vi "RT Buffered Logger.vi"(8 "error in (no error)":errorcluster, 11 "Logger Parameters":T1) -> (0 "error out":errorcluster, 3 "Logger Parameters":T1={"State"="", "Buffer size"=0, "Array Element size"=0, "Buffer Index"=0, "Data FIFO"=refnum, "is Shutdown"=FALSE, "Buffer"=[], "Log path"=path "C:/logs/AdvancedTDMS_Telemetry_Prototype.tdms", "File ref"=refnum, "Channel Names"=[]})   [LabVIEW 2019, in "Telemetry Engine.lvlib"]
uses:
  Telemetry Engine.lvlib
  Types/Logger Data.ctl
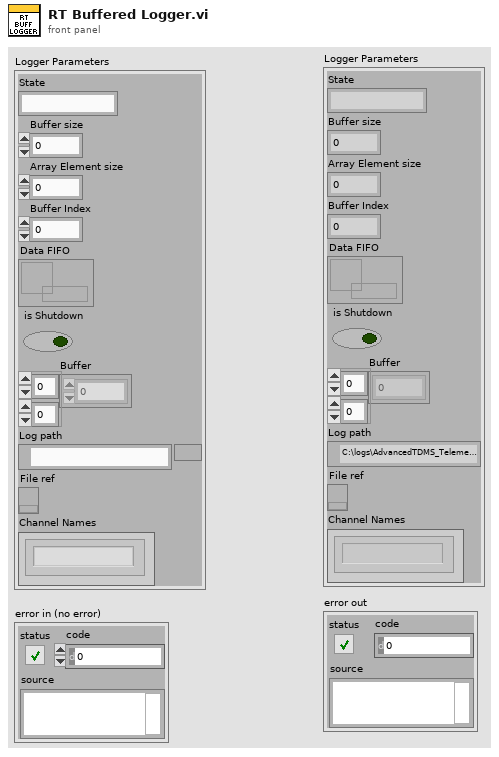
[diagram p1: front panel]
types:
  T1 = typedef "Telemetry Engine.lvlib/Logger Data.ctl" = cluster{"State":string, "Buffer size":i32, "Array Element size":i32, "Buffer Index":i32, "Data FIFO":refnum<k33>, "is Shutdown":bool, "Buffer":dbl[][], "Log path":path, "File ref":refnum<k34>, "Channel Names":string[]}
  T2 = enum16{"open", "open or create", "create or replace", "create", "open (read-only)"}
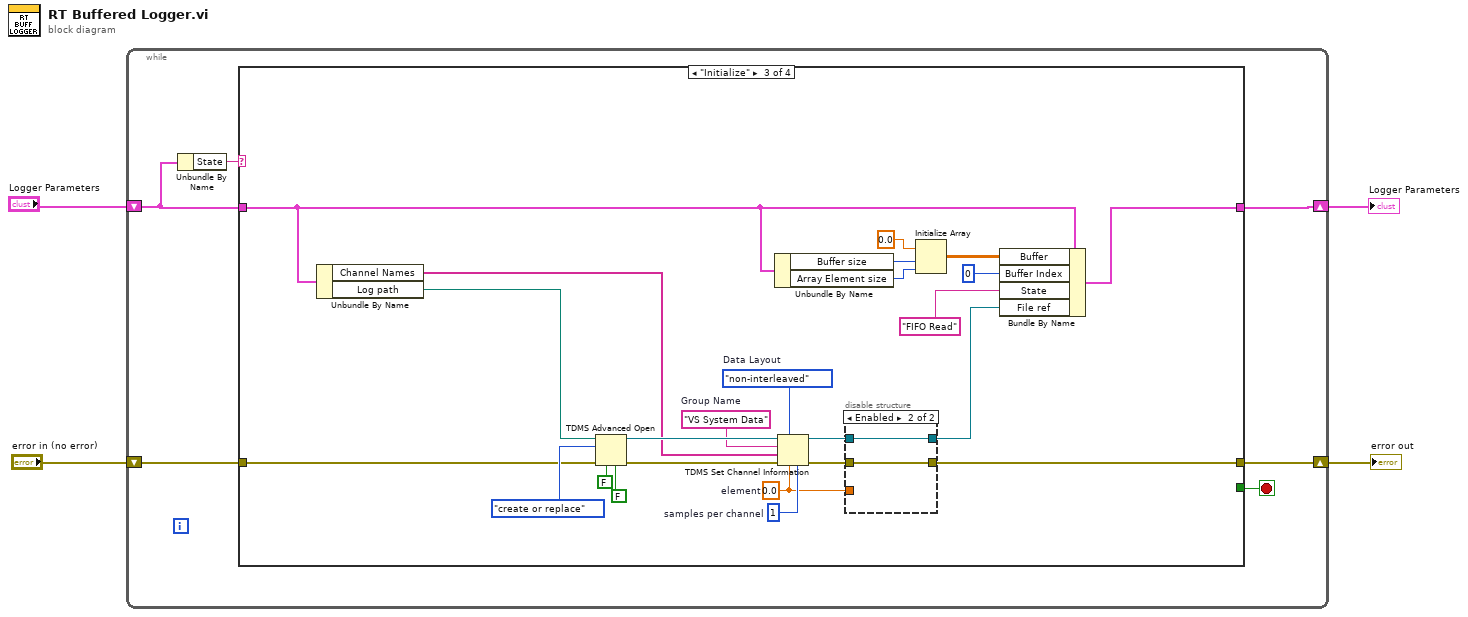
[diagram p0: block diagram]
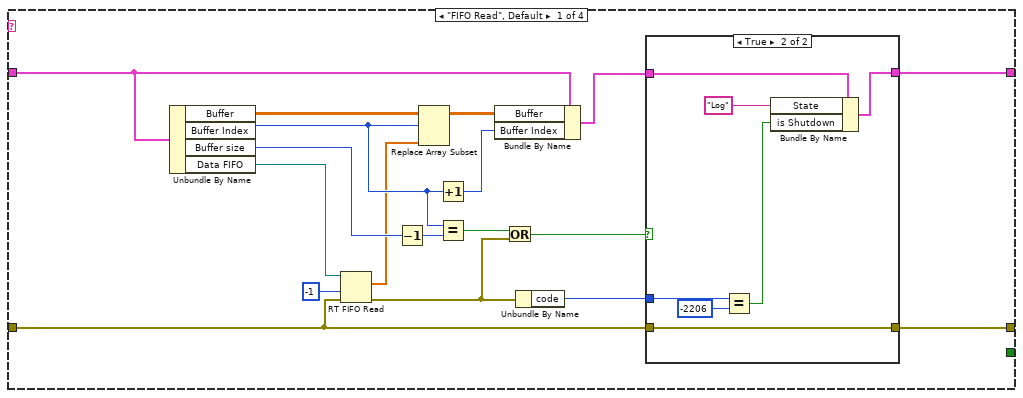
[diagram p2: hidden frame]
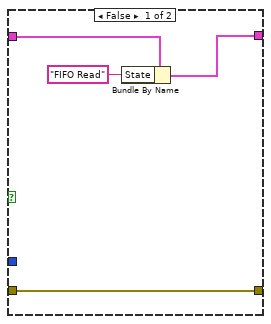
[diagram p3: hidden frame]
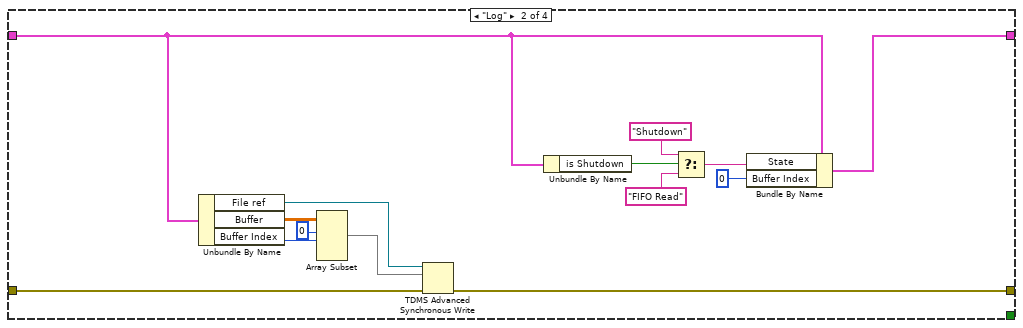
[diagram p4: hidden frame]
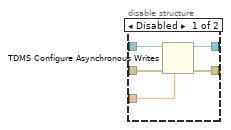
[diagram p5: hidden frame]
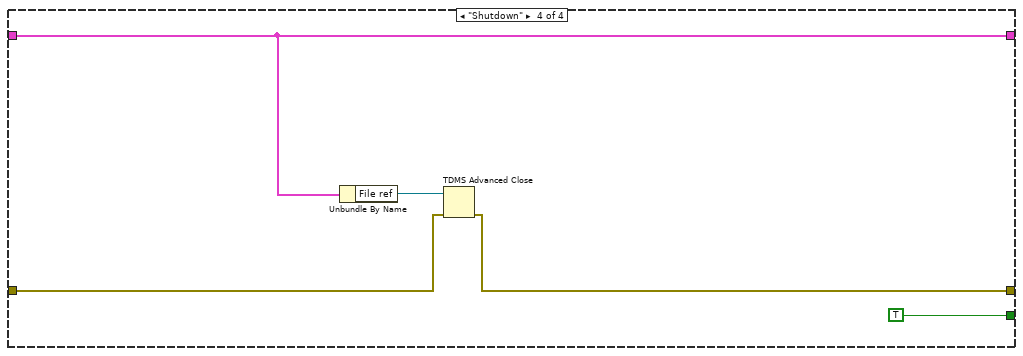
[diagram p6: hidden frame]
diagram:
  n1 = while {
    shift-right: [w9] -> w2
    shift-left: "Logger Parameters" -> [w8]
    shift-right: [w6] -> w1
    shift-left: "error in (no error)" -> [w5]
    stop <- w10 stop-if-true
    n2 = Unbundle By Name(w8) -> ("State"=w7:string)
    n3 = case shown="\"Initialize\"" w7 {
      tunnel: [_ _ _ TRUE] -> w10
      tunnel: w8 -> [w26 w46 w63 w88]
      tunnel: [w27 w51 w71 w88] -> w9
      tunnel: [w13 w42 w56 w85] -> w6
      tunnel: w5 -> [w14 w43 w55 w86]
      frame "FIFO Read", Default {
        n4 = Unbundle By Name(w26) -> ("Buffer"=w23:dbl[][], "Buffer Index"=w17:i32, "Buffer size"=w20:i32, "Data FIFO"=w12:refnum<k33>)
        n5 = RT FIFO Read(0:w12, 2:-1 ("timeout in ms (0)"), 3:w14) -> (9:w11:dbl[], 11:w16:errorcluster)  [unwired: 1 in, 3 out]
        n6 = Decrement(x=w20) -> (x-1=w19:i32)
        n7 = Replace Array Subset(array=w23, new element=w11, index (row)=w17) -> (w22:dbl[][])  [unwired: 1 in]
        n8 = Increment(x=w17) -> (x+1=w18:i32)
        n9 = Equal?(x=w17, y=w19) -> (x = y?=w25:bool)
        n10 = Bundle By Name(cluster=w26, "Buffer"=w22, "Buffer Index"=w18) -> (w21:T1)
        n11 = Or(x=w25, y=w16) -> (x .or. y?=w24:bool)
        n12 = Unbundle By Name(w16) -> ("code"=w15:i32)
        n13 = case shown="True" w24 {
          tunnel: w21 -> [w32 w39]
          tunnel: [w30 w38] -> w27
          tunnel: w15 -> [_ w37]
          tunnel: w14 -> [w29 w33]
          tunnel: [w29 w33] -> w13
          frame False {
            n14 = Bundle By Name(cluster=w32, "State"="FIFO Read") -> (w30:T1)
          }
          frame True {
            n15 = Equal?(x=w37, y=-2206) -> (x = y?=w35:bool)
            n16 = Bundle By Name(cluster=w39, "State"="Log", "is Shutdown"=w35) -> (w38:T1)
          }
        }
      }
      frame "Log" {
        n17 = Unbundle By Name(w46) -> ("File ref"=w41:refnum<k34>, "Buffer"=w44:dbl[][], "Buffer Index"=w45:i32)
        n18 = Array Subset(array=w44, index (row)=0 ("index"), length (row)=w45) -> (w40:dbl[][])  [unwired: 2 in]
        n19 = TDMS Advanced Synchronous Write(8:w43, 10:w40, 11:w41) -> (0:w42:errorcluster)  [unwired: 1 out]
        n20 = Unbundle By Name(w46) -> ("is Shutdown"=w50:bool)
        n21 = Select(t="Shutdown", s=w50, f="FIFO Read") -> (s? t:f=w47:string)
        n22 = Bundle By Name(cluster=w46, "State"=w47, "Buffer Index"=0 ("dimension size")) -> (w51:T1)
      }
      frame "Initialize" {
        w67 = enum16{"non-interleaved", "interleaved"}."non-interleaved"  # Data Layout
        w68 = u32 1  # samples per channel
        w58 = 0.0  # element
        w66 = "VS System Data"  # Group Name
        n23 = Unbundle By Name(w63) -> ("Channel Names"=w57:string[], "Log path"=w62:path)
        n24 = TDMS Advanced Open(4:FALSE ("enable asynchronous? (T)"), 6:FALSE ("disable buffering? (T)"), 8:w55, 10:T2."create or replace" ("operation (0:open)"), 11:w62) -> (0:w70:errorcluster, 3:w69:refnum<k34>)  [unwired: 1 out]
        n25 = Unbundle By Name(w63) -> ("Buffer size"=w77:i32, "Array Element size"=w75:i32)
        n26 = TDMS Set Channel Information(4:w68, 6:w58, 7:w67, 8:w70, 9:w57, 10:w66, 11:w69) -> (0:w60:errorcluster, 3:w61:refnum<k34>)
        n27 = disable-structure shown="Enabled" {
          disable-tunnel: w61 -> [w82 w84]
          disable-tunnel: w60 -> [w81 w83]
          disable-tunnel: [w80 w84] -> w59
          disable-tunnel: w58 -> [w79 _]
          disable-tunnel: [w78 w83] -> w56
          frame Disabled {
            n28 = TDMS Configure Asynchronous Writes(6:w79, 8:w81, 11:w82) -> (0:w78:errorcluster, 3:w80:refnum<k34>)  [unwired: 4 in]
          }
          frame Enabled {
          }
        }
        n29 = Initialize Array(0.0 ("element"), w77, w75) -> (w74:dbl[][])
        n30 = Bundle By Name(cluster=w63, "Buffer"=w74, "Buffer Index"=0, "State"="FIFO Read", "File ref"=w59) -> (w71:T1)
      }
      frame "Shutdown" {
        n31 = Unbundle By Name(w88) -> ("File ref"=w87:refnum<k34>)
        n32 = TDMS Advanced Close(8:w86, 11:w87) -> (0:w85:errorcluster)  [unwired: 2 in, 1 out]
      }
    }
  }
  "Logger Parameters" <- w2
  "error out" <- w1
